vi "Config info.vi"() -> (2 "info database local":T1, 6 "info database server":T3, 8 "info com main":T2)   [LabVIEW 2017]
uses:
  <vilib>/Utility/config.llb/Write Key (String).vi
  <vilib>/Utility/config.llb/Read Key (String).vi
  <vilib>/Utility/config.llb/NI_LVConfig.lvlib
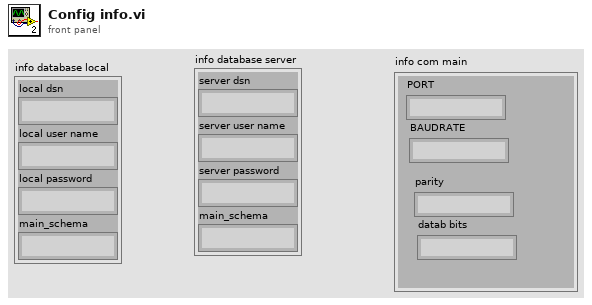
[diagram p1: front panel]
types:
  T1 = cluster{"local dsn":string, "local user name":string, "local password":string, "main_schema":string}
  T2 = cluster{"PORT":string, "BAUDRATE":string, "parity":string, "datab bits":string}
  T3 = cluster{"server dsn":string, "server user name":string, "server password":string, "main_schema":string}
  T4 = typedef "NI_LVConfig.lvlib/Config Data RefNum.ctl" = refnum<k1>
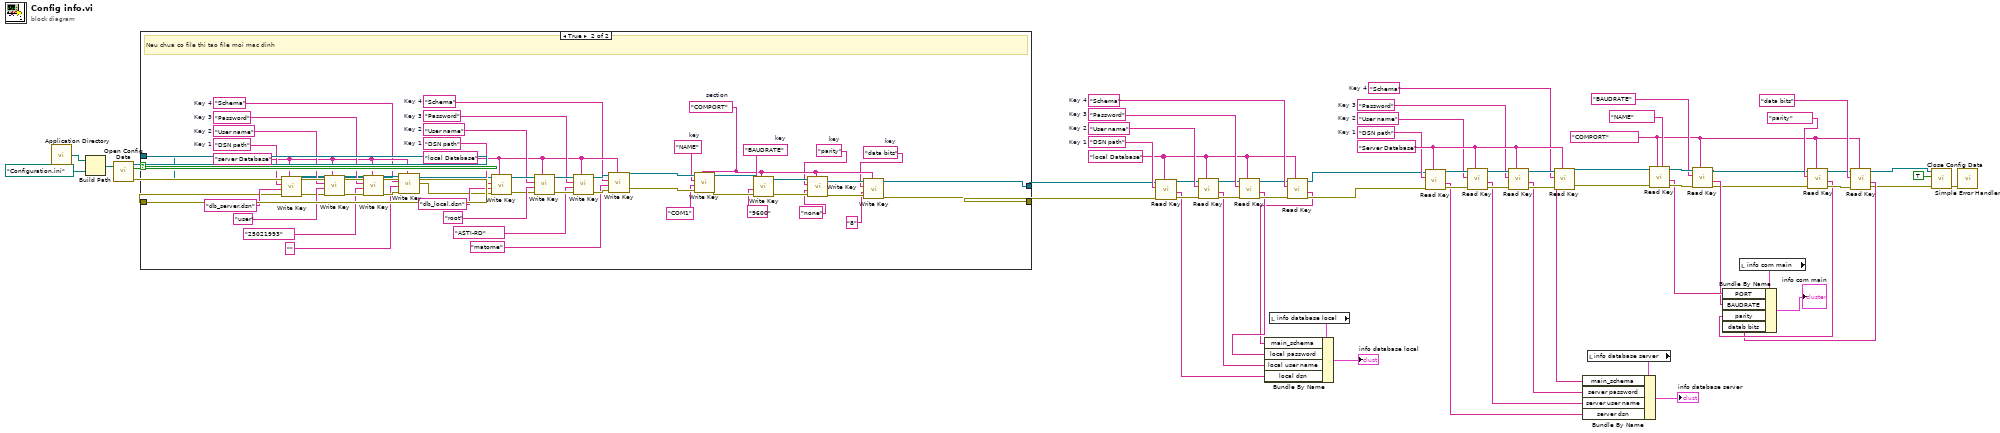
[diagram p0: block diagram]
diagram:
  w32 = "Schema"  # Key 4
  w31 = "Password"  # Key 3
  w30 = "User name"  # Key 2
  w29 = "DSN path"  # Key 1
  w28 = "local Database"
  w1 = "COMPORT" ("section")
  w49 = "Schema"  # Key 4
  w50 = "Password"  # Key 3
  w51 = "User name"  # Key 2
  w52 = "DSN path"  # Key 1
  w53 = "Server Database"
  n1 = call <vilib>:"Application Directory.vi"() -> ("Application Directory"=w56:path)
  n2 = Build Path(base path=w56, name or relative path=path "Configuration.ini" ("default name")) -> (appended path=w66:path)
  n3 = call <vilib>:"Open Config Data.vi"("configuration file path"=w66) -> ("error out"=w64:errorcluster, "file created?"=w61:bool, "refnum"=w65:T4)  [unwired: 2 in, 6 out]
  n4 = case shown="True" w61 {
    tunnel: w65 -> [w69 w82]
    tunnel: w64 -> [w68 w81]
    tunnel: [w69 w71] -> w19
    tunnel: [w68 w70] -> w18
    frame False {
    }
    frame True {
      w75 = "data bits"  # key
      w76 = "parity"  # key
      w87 = "Schema"  # Key 4
      w93 = "Password"  # Key 3
      w92 = "User name"  # Key 2
      w91 = "DSN path"  # Key 1
      w88 = "server Database"
      w104 = "BAUDRATE"  # key
      w105 = "NAME"  # key
      w77 = "COMPORT"  # section
      w110 = "Schema"  # Key 4
      w116 = "Password"  # Key 3
      w115 = "User name"  # Key 2
      w114 = "DSN path"  # Key 1
      w111 = "local Database"
      # "Neu chua co file thi tao file moi mac dinh"
      n5 = call-poly <vilib>:"Write Key.vi"("section"=w88, "error in (no error)"=w81, "value"="db_server.dsn", "key"=w91, "refnum"=w82) -> ("error out"=w94:errorcluster, "refnum out"=w95:T4)  [unwired: 4 in, 1 out]
      n6 = call-poly <vilib>:"Write Key.vi"("section"=w88, "error in (no error)"=w94, "value"="user", "key"=w92, "refnum"=w95) -> ("error out"=w99:errorcluster, "refnum out"=w98:T4)  [unwired: 1 in, 4 out]
      n7 = call-poly <vilib>:"Write Key.vi"("section"=w88, "error in (no error)"=w99, "value"="25021993", "key"=w93, "refnum"=w98) -> ("error out"=w90:errorcluster, "refnum out"=w89:T4)  [unwired: 1 in, 4 out]
      n8 = call-poly <vilib>:"Write Key.vi"("section"=w88, "error in (no error)"=w90, "value"="", "key"=w87, "refnum"=w89) -> ("error out"=w83:errorcluster, "refnum out"=w84:T4)  [unwired: 1 in, 4 out]
      n9 = call-poly <vilib>:"Write Key.vi"("section"=w111, "error in (no error)"=w83, "value"="db_local.dsn", "key"=w114, "refnum"=w84) -> ("error out"=w117:errorcluster, "refnum out"=w118:T4)  [unwired: 4 in, 1 out]
      n10 = call-poly <vilib>:"Write Key.vi"("section"=w111, "error in (no error)"=w117, "value"="root", "key"=w115, "refnum"=w118) -> ("error out"=w122:errorcluster, "refnum out"=w121:T4)  [unwired: 1 in, 4 out]
      n11 = call-poly <vilib>:"Write Key.vi"("section"=w111, "error in (no error)"=w122, "value"="ASTI-RD", "key"=w116, "refnum"=w121) -> ("error out"=w113:errorcluster, "refnum out"=w112:T4)  [unwired: 1 in, 4 out]
      n12 = call-poly <vilib>:"Write Key.vi"("section"=w111, "error in (no error)"=w113, "value"="matome", "key"=w110, "refnum"=w112) -> ("error out"=w107:errorcluster, "refnum out"=w106:T4)  [unwired: 1 in, 4 out]
      n13 = call-poly <vilib>:"Write Key.vi"("section"=w77, "error in (no error)"=w107, "value"="COM1", "key"=w105, "refnum"=w106) -> ("error out"=w102:errorcluster, "refnum out"=w103:T4)  [unwired: 1 in, 4 out]
      n14 = call-poly <vilib>:"Write Key.vi"("section"=w77, "error in (no error)"=w102, "value"="9600", "key"=w104, "refnum"=w103) -> ("error out"=w78:errorcluster, "refnum out"=w79:T4)  [unwired: 1 in, 4 out]
      n15 = call-poly <vilib>:"Write Key.vi"("section"=w77, "error in (no error)"=w78, "value"="none", "key"=w76, "refnum"=w79) -> ("error out"=w74:errorcluster, "refnum out"=w80:T4)  [unwired: 1 in, 4 out]
      n16 = call-poly <vilib>:"Write Key.vi"("section"=w77, "error in (no error)"=w74, "value"="8", "key"=w75, "refnum"=w80) -> ("error out"=w70:errorcluster, "refnum out"=w71:T4)  [unwired: 1 in, 4 out]
    }
  }
  n17 = call-poly <vilib>:"Read Key.vi"("section"=w28, "error in (no error)"=w18, "key"=w29, "refnum"=w19) -> ("error out"=w23:errorcluster, "value"=w15:string, "refnum out"=w22:T4)  [unwired: 4 in, 1 out]
  n18 = call-poly <vilib>:"Read Key.vi"("section"=w28, "error in (no error)"=w23, "key"=w30, "refnum"=w22) -> ("error out"=w24:errorcluster, "value"=w14:string, "refnum out"=w25:T4)  [unwired: 2 in, 3 out]
  n19 = call-poly <vilib>:"Read Key.vi"("section"=w28, "error in (no error)"=w24, "key"=w31, "refnum"=w25) -> ("error out"=w27:errorcluster, "value"=w13:string, "refnum out"=w26:T4)  [unwired: 2 in, 3 out]
  n20 = local read "info database local"() -> (w16:T1)
  n21 = call-poly <vilib>:"Read Key.vi"("section"=w28, "error in (no error)"=w27, "key"=w32, "refnum"=w26) -> ("error out"=w20:errorcluster, "value"=w12:string, "refnum out"=w21:T4)  [unwired: 2 in, 3 out]
  n22 = Bundle By Name(cluster=w16, "main_schema"=w12, "local password"=w13, "local user name"=w14, "local dsn"=w15) -> (→"info database local":T1)
  n23 = call-poly <vilib>:"Read Key.vi"("section"=w53, "error in (no error)"=w20, "key"=w52, "refnum"=w21) -> ("error out"=w59:errorcluster, "value"=w46:string, "refnum out"=w60:T4)  [unwired: 4 in, 1 out]
  n24 = call-poly <vilib>:"Read Key.vi"("section"=w53, "error in (no error)"=w59, "key"=w51, "refnum"=w60) -> ("error out"=w58:errorcluster, "value"=w45:string, "refnum out"=w57:T4)  [unwired: 2 in, 3 out]
  n25 = call-poly <vilib>:"Read Key.vi"("section"=w53, "error in (no error)"=w58, "key"=w50, "refnum"=w57) -> ("error out"=w54:errorcluster, "value"=w44:string, "refnum out"=w55:T4)  [unwired: 2 in, 3 out]
  n26 = call-poly <vilib>:"Read Key.vi"("section"=w53, "error in (no error)"=w54, "key"=w49, "refnum"=w55) -> ("error out"=w39:errorcluster, "value"=w43:string, "refnum out"=w41:T4)  [unwired: 2 in, 3 out]
  n27 = local read "info database server"() -> (w48:T3)
  n28 = Bundle By Name(cluster=w48, "main_schema"=w43, "server password"=w44, "server user name"=w45, "server dsn"=w46) -> (→"info database server":T3)
  n29 = call-poly <vilib>:"Read Key.vi"("section"=w1, "error in (no error)"=w39, "key"="NAME", "refnum"=w41) -> ("error out"=w40:errorcluster, "value"=w34:string, "refnum out"=w42:T4)  [unwired: 2 in, 3 out]
  n30 = call-poly <vilib>:"Read Key.vi"("section"=w1, "error in (no error)"=w40, "key"="BAUDRATE", "refnum"=w42) -> ("error out"=w6:errorcluster, "value"=w33:string, "refnum out"=w7:T4)  [unwired: 2 in, 3 out]
  n31 = local read "info com main"() -> (w35:T2)
  n32 = call-poly <vilib>:"Read Key.vi"("section"=w1, "error in (no error)"=w6, "key"="parity", "refnum"=w7) -> ("error out"=w9:errorcluster, "value"=w5:string, "refnum out"=w8:T4)  [unwired: 2 in, 3 out]
  n33 = call-poly <vilib>:"Read Key.vi"("section"=w1, "error in (no error)"=w9, "key"="data bits", "refnum"=w8) -> ("error out"=w2:errorcluster, "value"=w4:string, "refnum out"=w3:T4)  [unwired: 2 in, 3 out]
  n34 = Bundle By Name(cluster=w35, "PORT"=w34, "BAUDRATE"=w33, "parity"=w5, "datab bits"=w4) -> (→"info com main":T2)
  n35 = call <vilib>:"Close Config Data.vi"("error in (no error)"=w2, "write file if changed (T)"=TRUE ("write configuration file? (T)"), "refnum"=w3) -> ("error out"=w63:errorcluster)  [unwired: 8 out]
  n36 = call <vilib>:"Simple Error Handler.vi"("error in (no error)"=w63) -> ()  [unwired: 1 in, 8 out]
